vi "_9For_Loop.vi"() -> ()   [LabVIEW 2018]
panel:
  out "?":dbl
  in  "?":dbl
  # "Sum Of N Terms"
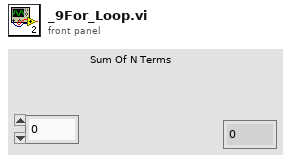
[diagram p1: front panel]
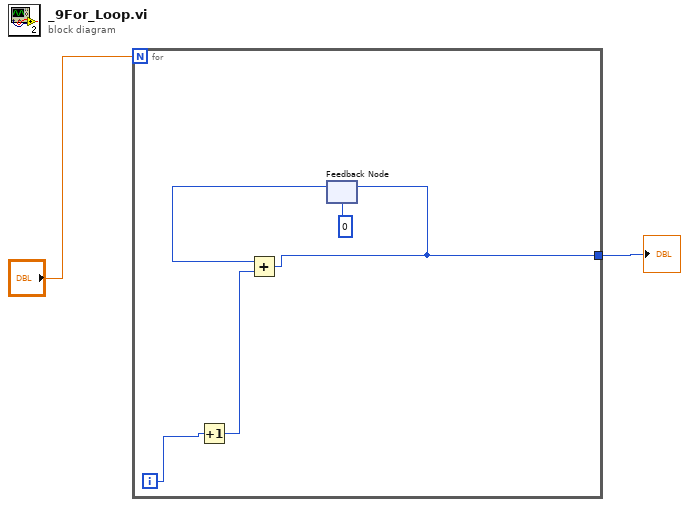
[diagram p0: block diagram]
diagram:
  n1 = for {
    N: "?" -> [_]
    tunnel: [w3] -> w1
    i -> [w7]
    n2 = Increment(x=w7) -> (x+1=w6:i32)
    n3 = feedback #1(0) -> (w5:i32)
    n4 = Add(x=w5, y=w6) -> (x+y=w3:i32)
    n5 = feedback-in #1(w3) -> ()
  }
  "?" <- w1
